vi "Write Payload.vi"(8 "error in (no error)":errorcluster, 10 "uData.lvlib:uData.lvclass":refnum<class "uData.lvclass">, 11 "uMsg in":refnum<class "uMsg.lvclass">) -> (0 "error out":errorcluster, 3 "uMsg out":refnum<class "uMsg.lvclass">)   [LabVIEW 2023, in "uLib.lvlib" / "uMsg.lvclass"]
uses:
  uMsg.lvclass
  uData/uData/uData.lvclass
  uMsg.lvclass/uMsg.ctl
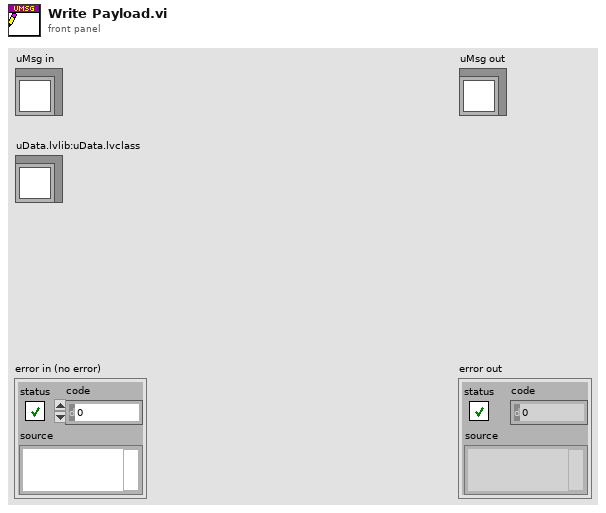
[diagram p1: front panel]
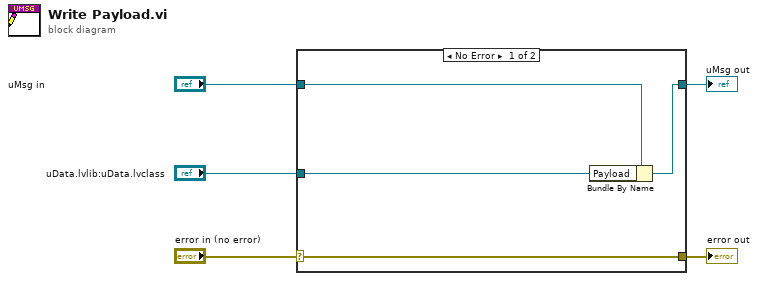
[diagram p0: block diagram]
diagram:
  n1 = case shown="No Error" "error in (no error)" {
    selector: "error in (no error)" -> [w9 w10]
    tunnel: [w9 w10] -> w4
    tunnel: [w7 w11] -> w2
    tunnel: "uMsg in" -> [w8 w11]
    tunnel: "uData.lvlib:uData.lvclass" -> [w6 _]
    frame No Error {
      n2 = Bundle By Name(cluster=w8, "Payload"=w6) -> (w7:refnum<class "uMsg.lvclass">)
    }
    frame Error {
    }
  }
  "error out" <- w4
  "uMsg out" <- w2
